vi "Startup Dialog.vi"(8 "error in":errorcluster) -> (0 "error out":errorcluster, 3 "appended path":path)   [LabVIEW 2025, in "I2C Bus Monitor UI.lvlib"]
uses:
  I2C Bus Monitor UI.lvlib
  <vilib>/Utility/config.llb/Read Key (Boolean).vi
  Error Global.vi
  <vilib>/Utility/config.llb/Write Key (Boolean).vi
  <vilib>/Utility/config.llb/NI_LVConfig.lvlib
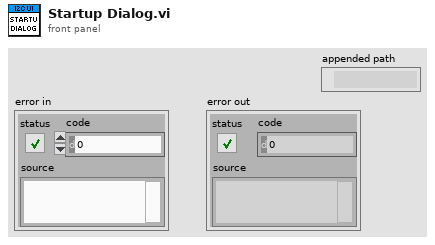
[diagram p1: front panel]
types:
  T1 = typedef "NI_LVConfig.lvlib/Config Data RefNum.ctl" = refnum<k1>
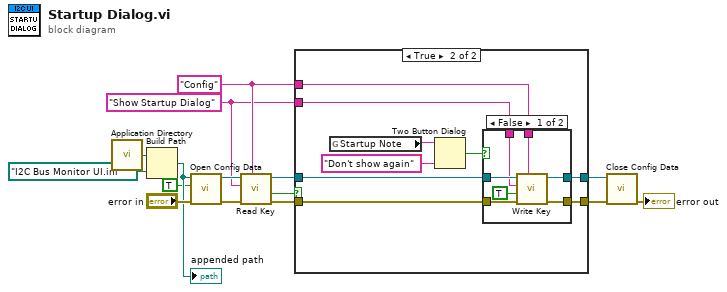
[diagram p0: block diagram]
diagram:
  w3 = "Config" ("section")
  w2 = "Show Startup Dialog" ("key")
  n1 = call <vilib>:"Application Directory.vi"() -> ("Application Directory"=w1:path)
  n2 = Build Path(base path=w1, name or relative path=path "I2C Bus Monitor UI.ini") -> (appended path=w12:path)
  "appended path" <- w12
  n3 = call <vilib>:"Open Config Data.vi"("error in (no error)"="error in", "create file if necessary (T)"=TRUE, "configuration file path"=w12) -> ("error out"=w11:errorcluster, "refnum"=w10:T1)  [unwired: 6 in, 1 out]
  n4 = call-poly <vilib>:"Read Key.vi"("section"=w3, "error in (no error)"=w11, "key"=w2, "refnum"=w10) -> ("error out"=w8:errorcluster, "value"=w7:bool, "refnum out"=w6:T1)  [unwired: 4 in, 1 out]
  n5 = case shown="True" w7 {
    tunnel: [w17 w26] -> w14
    tunnel: w8 -> [w17 w25]
    tunnel: w6 -> [w16 w21]
    tunnel: [w16 w20] -> w4
    tunnel: w3 -> [_ w19]
    tunnel: w2 -> [_ w18]
    frame False {
    }
    frame True {
      n6 = global read "Error Global.vi" "Startup Note"() -> (w24:string)
      n7 = Two Button Dialog(message=w24, 1:"Don't show again" ("F button name (\"Cancel\")")) -> (T button?=w22:bool)  [unwired: 1 in]
      n8 = case shown="False" w22 {
        tunnel: [w32 w35] -> w26
        tunnel: w25 -> [w33 w35]
        tunnel: w21 -> [w31 w34]
        tunnel: [w30 w34] -> w20
        tunnel: w19 -> [w29 _]
        tunnel: w18 -> [w28 _]
        frame False {
          n9 = call-poly <vilib>:"Write Key.vi"("section"=w29, "error in (no error)"=w33, "value"=TRUE, "key"=w28, "refnum"=w31) -> ("error out"=w32:errorcluster, "refnum out"=w30:T1)  [unwired: 4 in, 1 out]
        }
        frame True {
        }
      }
    }
  }
  n10 = call <vilib>:"Close Config Data.vi"("error in (no error)"=w14, "refnum"=w4) -> ("error out"=→"error out":errorcluster)  [unwired: 8 in, 1 out]
